vi "ep_Check Nameplate (Load).vi"(8 "error in (no error)":errorcluster, 11 "nameplate information":T1) -> (0 "error out":errorcluster, 2 "full load efficiency [%]":dbl)   [LabVIEW 2014, in "NI_EP_Motor Monitoring.lvlib"]
uses:
  <vilib>/addons/Electrical Power/Motor Monitoring/NI_EP_Motor Monitoring.lvlib
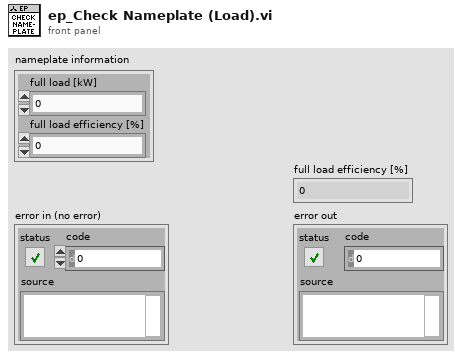
[diagram p1: front panel]
types:
  T1 = cluster{"full load [kW]":dbl, "full load efficiency [%]":dbl}
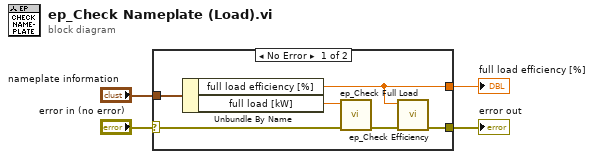
[diagram p0: block diagram]
diagram:
  n1 = case shown="No Error" "error in (no error)" {
    selector: "error in (no error)" -> [w8 w11]
    tunnel: [w6 w11] -> w2
    tunnel: "nameplate information" -> [w10 _]
    tunnel: [w5 _] -> w1
    frame No Error {
      n2 = Unbundle By Name(w10) -> ("full load efficiency [%]"=w5:dbl, "full load [kW]"=w9:dbl)
      n3 = call <vilib>:"ep_Check Full Load.vi"("error in (no error)"=w8, "full load [W]"=w9) -> ("error out"=w7:errorcluster)  [unwired: 9 in]
      n4 = call <vilib>:"ep_Check Efficiency.vi"("error in (no error)"=w7, "efficiency [%]"=w5) -> ("error out"=w6:errorcluster)  [unwired: 9 in]
    }
    frame Error {
    }
  }
  "error out" <- w2
  "full load efficiency [%]" <- w1
